vi "SQL_test_data_insert.vi"(10 "通道名":T1={"声发射", "电涡流1", "电涡流2", "电涡流3", "电涡流4", "电涡流5", "加速度1", "加速度2"}, 11 "数据":T2={"时间"=timestamp(3515985789.500352 s since 1904-01-01), "声发射"=array[32000 elements], "电涡流1"=array[32000 elements], "电涡流2"=array[32000 elements], "电涡流3"=array[32000 elements], "电涡流4"=array[32000 elements], "电涡流5"=array[32000 elements], "加速度1"=array[80000 elements], "加速度2"=array[80000 elements]}) -> (2 "数据插入时间ms":u32, 3 "error out":errorcluster)   [LabVIEW 2014]
uses:
  <vilib>/addons/database/Connection.llb/DB Tools Open Connec (String).vi
  <vilib>/addons/database/Connection.llb/Conn Execute.vi
  <vilib>/addons/database/Recordset.llb/Rec Destroy - Connection.vi
  <vilib>/addons/database/NI_Database_API.lvlib
panel:
  out "x-y":u32
  out "毫秒计时值 2":u32
  out "毫秒计时值":u32
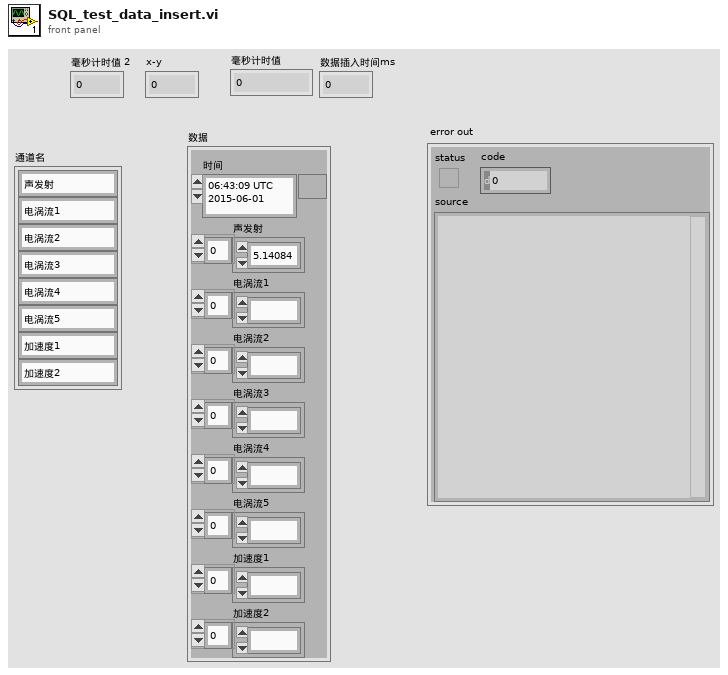
[diagram p1: front panel]
types:
  T1 = cluster{string, string, string, string, string, string, string, string}
  T2 = cluster{"时间":timestamp, "声发射":sgl[], "电涡流1":sgl[], "电涡流2":sgl[], "电涡流3":sgl[], "电涡流4":sgl[], "电涡流5":sgl[], "加速度1":sgl[], "加速度2":sgl[]}
  T3 = typedef "NI_Database_API.lvlib/Conn ObjectReference.ctl" = refnum<k1>
  T4 = typedef "NI_Database_API.lvlib/Rec ObjectReference.ctl" = refnum<k1>
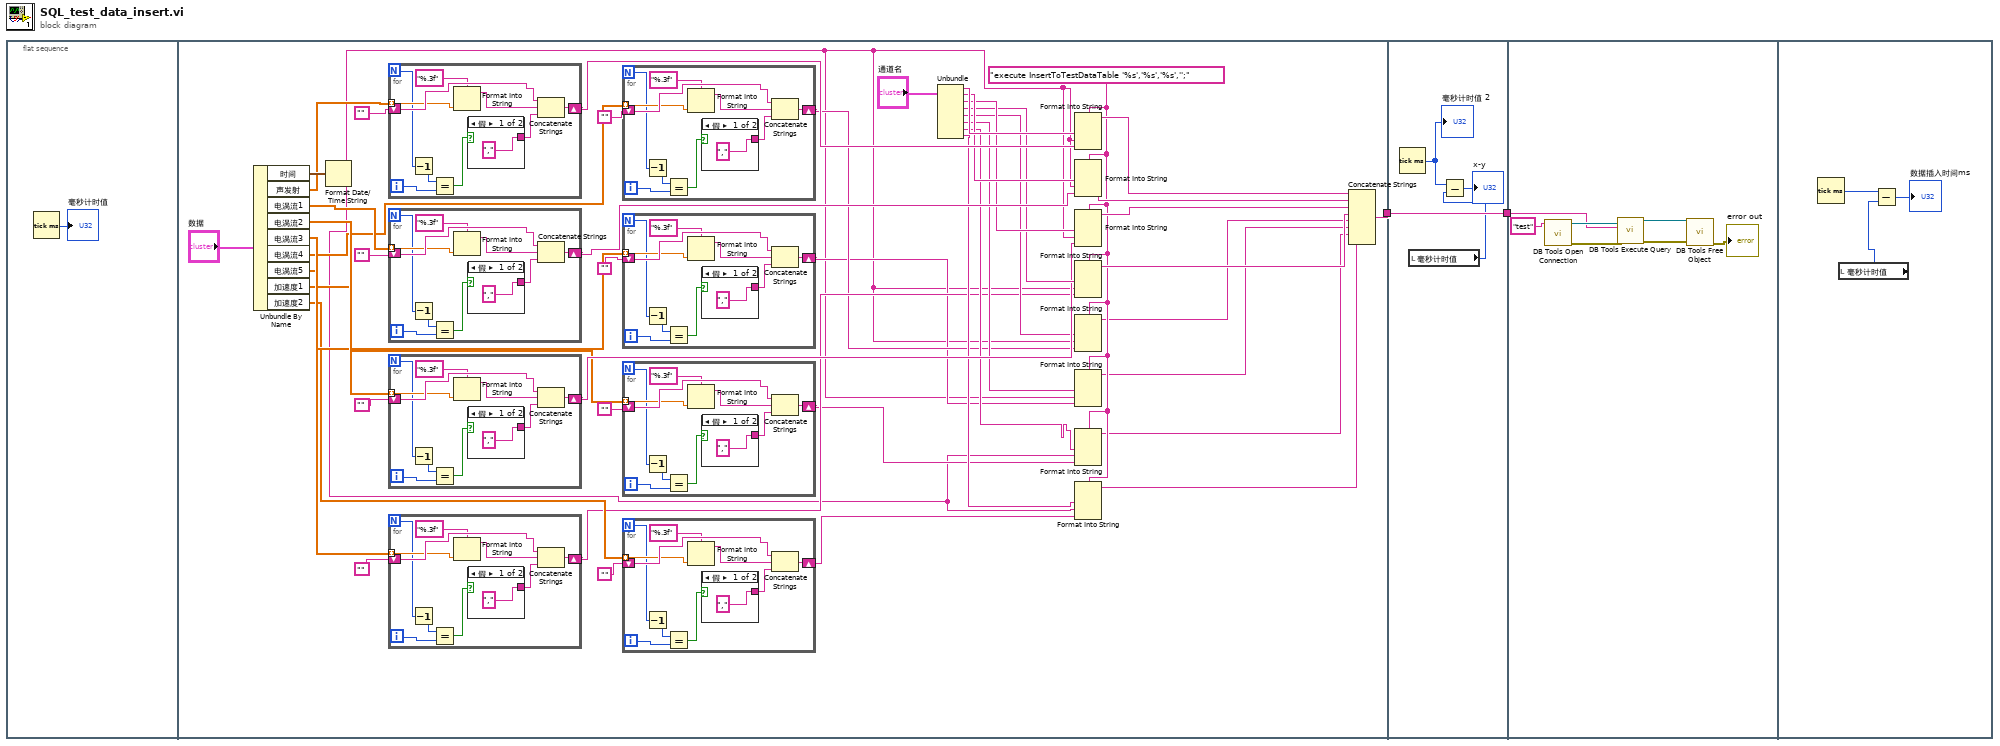
[diagram p0: block diagram]
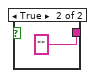
[diagram p2: hidden frame]
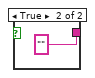
[diagram p3: hidden frame]
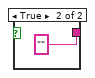
[diagram p4: hidden frame]
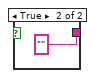
[diagram p5: hidden frame]
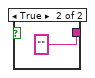
[diagram p6: hidden frame]
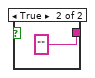
[diagram p7: hidden frame]
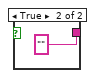
[diagram p8: hidden frame]
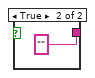
[diagram p9: hidden frame]
diagram:
  n1 = flat-sequence {
    tunnel: [w49] -> w2
    tunnel: w2 -> [w149]
    tunnel: [w149] -> w1
    tunnel: w1 -> [w150]
    frame #0 {
      n2 = Tick Count (ms)() -> (millisecond timer value=→"毫秒计时值":u32)
    }
    frame #1 {
      w14 = "execute InsertToTestDataTable '%s','%s','%s','';"
      n3 = Unbundle By Name("数据") -> ("时间"=w48:timestamp, "声发射"=w42:sgl[], "电涡流1"=w41:sgl[], "电涡流2"=w39:sgl[], "电涡流3"=w37:sgl[], "电涡流4"=w26:sgl[], "电涡流5"=w25:sgl[], "加速度1"=w24:sgl[], "加速度2"=w23:sgl[])
      n4 = Format Date/Time String(seconds (now)=w48) -> (date/time string=w8:string)  [unwired: 2 in]
      n5 = for "For循环" {
        N -> [w136]
        tunnel: w42 -> [w141] mode=indexing
        shift-right: [w142] -> w45
        shift-left: "" -> [w143]
        i -> [w138]
        n6 = Decrement(x=w136) -> (x-1=w137:i32)
        n7 = Equal?(x=w137, y=w138) -> (x = y?=w135:bool)
        n8 = Format Into String(format string="%.3f", w141) -> (resulting string=w140:string)  [unwired: 2 in, 1 out]
        n9 = case shown="假" w135 {
          tunnel: ["," ""] -> w134
          frame False {
          }
          frame True {
          }
        }
        n10 = Concatenate Strings(w143, w140, w134) -> (w142:string)
      }
      n11 = for "For循环" {
        N -> [w124]
        tunnel: w41 -> [w129] mode=indexing
        shift-right: [w130] -> w35
        shift-left: "" -> [w131]
        i -> [w126]
        n12 = Decrement(x=w124) -> (x-1=w125:i32)
        n13 = Equal?(x=w125, y=w126) -> (x = y?=w123:bool)
        n14 = Format Into String(format string="%.3f", w129) -> (resulting string=w128:string)  [unwired: 2 in, 1 out]
        n15 = case shown="假" w123 {
          tunnel: ["," ""] -> w122
          frame False {
          }
          frame True {
          }
        }
        n16 = Concatenate Strings(w131, w128, w122) -> (w130:string)
      }
      n17 = for "For循环" {
        N -> [w112]
        tunnel: w39 -> [w117] mode=indexing
        shift-right: [w118] -> w30
        shift-left: "" -> [w119]
        i -> [w114]
        n18 = Decrement(x=w112) -> (x-1=w113:i32)
        n19 = Equal?(x=w113, y=w114) -> (x = y?=w111:bool)
        n20 = Format Into String(format string="%.3f", w117) -> (resulting string=w116:string)  [unwired: 2 in, 1 out]
        n21 = case shown="假" w111 {
          tunnel: ["," ""] -> w110
          frame False {
          }
          frame True {
          }
        }
        n22 = Concatenate Strings(w119, w116, w110) -> (w118:string)
      }
      n23 = for "For循环" {
        N -> [w100]
        tunnel: w37 -> [w105] mode=indexing
        shift-right: [w106] -> w13
        shift-left: "" -> [w107]
        i -> [w102]
        n24 = Decrement(x=w100) -> (x-1=w101:i32)
        n25 = Equal?(x=w101, y=w102) -> (x = y?=w99:bool)
        n26 = Format Into String(format string="%.3f", w105) -> (resulting string=w104:string)  [unwired: 2 in, 1 out]
        n27 = case shown="假" w99 {
          tunnel: ["," ""] -> w98
          frame False {
          }
          frame True {
          }
        }
        n28 = Concatenate Strings(w107, w104, w98) -> (w106:string)
      }
      n29 = for "For循环" {
        N -> [w88]
        tunnel: w26 -> [w93] mode=indexing
        shift-right: [w94] -> w12
        shift-left: "" -> [w95]
        i -> [w90]
        n30 = Decrement(x=w88) -> (x-1=w89:i32)
        n31 = Equal?(x=w89, y=w90) -> (x = y?=w87:bool)
        n32 = Format Into String(format string="%.3f", w93) -> (resulting string=w92:string)  [unwired: 2 in, 1 out]
        n33 = case shown="假" w87 {
          tunnel: ["," ""] -> w86
          frame False {
          }
          frame True {
          }
        }
        n34 = Concatenate Strings(w95, w92, w86) -> (w94:string)
      }
      n35 = for "For循环" {
        N -> [w76]
        tunnel: w25 -> [w81] mode=indexing
        shift-right: [w82] -> w11
        shift-left: "" -> [w83]
        i -> [w78]
        n36 = Decrement(x=w76) -> (x-1=w77:i32)
        n37 = Equal?(x=w77, y=w78) -> (x = y?=w75:bool)
        n38 = Format Into String(format string="%.3f", w81) -> (resulting string=w80:string)  [unwired: 2 in, 1 out]
        n39 = case shown="假" w75 {
          tunnel: ["," ""] -> w74
          frame False {
          }
          frame True {
          }
        }
        n40 = Concatenate Strings(w83, w80, w74) -> (w82:string)
      }
      n41 = for "For循环" {
        N -> [w64]
        tunnel: w24 -> [w69] mode=indexing
        shift-right: [w70] -> w10
        shift-left: "" -> [w71]
        i -> [w66]
        n42 = Decrement(x=w64) -> (x-1=w65:i32)
        n43 = Equal?(x=w65, y=w66) -> (x = y?=w63:bool)
        n44 = Format Into String(format string="%.3f", w69) -> (resulting string=w68:string)  [unwired: 2 in, 1 out]
        n45 = case shown="假" w63 {
          tunnel: ["," ""] -> w62
          frame False {
          }
          frame True {
          }
        }
        n46 = Concatenate Strings(w71, w68, w62) -> (w70:string)
      }
      n47 = for "For循环" {
        N -> [w52]
        tunnel: w23 -> [w57] mode=indexing
        shift-right: [w58] -> w9
        shift-left: "" -> [w59]
        i -> [w54]
        n48 = Decrement(x=w52) -> (x-1=w53:i32)
        n49 = Equal?(x=w53, y=w54) -> (x = y?=w51:bool)
        n50 = Format Into String(format string="%.3f", w57) -> (resulting string=w56:string)  [unwired: 2 in, 1 out]
        n51 = case shown="假" w51 {
          tunnel: ["," ""] -> w50
          frame False {
          }
          frame True {
          }
        }
        n52 = Concatenate Strings(w59, w56, w50) -> (w58:string)
      }
      n53 = Unbundle("通道名") -> (w34:string, w33:string, w32:string, w31:string, w18:string, w17:string, w16:string, w15:string)
      n54 = Format Into String ("格式化写入字符串")(format string=w14, w34, w8, w45) -> (resulting string=w47:string)  [unwired: 2 in, 1 out]
      n55 = Format Into String ("格式化写入字符串")(format string=w14, w33, w8, w35) -> (resulting string=w29:string)  [unwired: 2 in, 1 out]
      n56 = Format Into String ("格式化写入字符串")(format string=w14, w32, w8, w30) -> (resulting string=w28:string)  [unwired: 2 in, 1 out]
      n57 = Format Into String ("格式化写入字符串")(format string=w14, w31, w8, w13) -> (resulting string=w27:string)  [unwired: 2 in, 1 out]
      n58 = Format Into String ("格式化写入字符串")(format string=w14, w18, w8, w12) -> (resulting string=w7:string)  [unwired: 2 in, 1 out]
      n59 = Format Into String ("格式化写入字符串")(format string=w14, w17, w8, w11) -> (resulting string=w6:string)  [unwired: 2 in, 1 out]
      n60 = Format Into String ("格式化写入字符串")(format string=w14, w16, w8, w10) -> (resulting string=w5:string)  [unwired: 2 in, 1 out]
      n61 = Format Into String ("格式化写入字符串")(format string=w14, w15, w8, w9) -> (resulting string=w4:string)  [unwired: 2 in, 1 out]
      n62 = Concatenate Strings ("连接字符串")(w47, w29, w28, w27, w7, w6, w5, w4) -> (w49:string)
    }
    frame #2 {
      n63 = Tick Count (ms)() -> (millisecond timer value=w148:u32)
      "毫秒计时值 2" <- w148
      n64 = local read "毫秒计时值"() -> (w147:u32)
      n65 = Subtract(x=w148, y=w147) -> (x-y=→"x-y":u32)
    }
    frame #3 {
      n66 = call-poly <vilib>:"DB Tools Open Connection.vi"("connection information"="test") -> ("error out"=w156:errorcluster, "connection reference"=w155:T3)  [unwired: 7 in]
      n67 = call-poly <vilib>:"DB Tools Execute Query.vi"("error in (no error)"=w156, "SQL query"=w150, "connection reference"=w155) -> ("error out"=w153:errorcluster, "recordset reference"=w152:T4)  [unwired: 5 in]
      n68 = call-poly <vilib>:"DB Tools Free Object.vi"("error in (no error)"=w153, "recordset reference"=w152) -> ("error out"=→"error out":errorcluster)  [unwired: 8 in, 1 out]
    }
    frame #4 {
      n69 = Tick Count (ms)() -> (millisecond timer value=w159:u32)
      n70 = local read "毫秒计时值"() -> (w157:u32)
      n71 = Subtract(x=w159, y=w157) -> (x-y=→"数据插入时间ms":u32)
    }
  }
